vi "Kart_Pv_Emulator.vi"() -> ()   [LabVIEW 2016]
uses:
  <vilib>/Instr/_visa.llb/VISA Configure Serial Port (Instr).vi
  <vilib>/Utility/file.llb/Read From Spreadsheet File (DBL).vi
panel:
  out "error out":errorcluster
  out "Döngü Time":u32
  out "Veriler Grafiği":T1(graph)
  out "Model_I":dbl
  out "Model_V":dbl
  out "e_I":dbl
  out "e_V":dbl
  out "NuData":i32
  out "GucK_R":dbl
  out "PgucK":dbl=60.0
  out "Vi Panel":dbl
  out "GucK_W":dbl(knob) scale=0.0..60.0
  out "GucK_V":dbl(knob) scale=0.0..22.0
  in  "Port Sec":refnum<visa-resource-name>="COM1"
  out "GucK_I":dbl(knob) scale=0.0..3.7
  out "10_dk_ok":bool
  out "time":dbl
  out "i_Data":i32
  out "File patch":path
  out "Güç Grafiği":cluster{"PmaxM":dbl, "Pmaxe":dbl, "PgucK":dbl}(graph)
  in  "a":dbl=110.681443442253
  in  "Rs":dbl=25.0
  out "M_Pmax":dbl=60.29985558543294
  out "V - I Grafiği":cluster{"Vi":dbl, "Iint":dbl, dbl}(graph)={"Vi"=21.500000000000036, "Iint"=0.07178993987123095, 1.5434837072314678}
  in  "Rsh":dbl=110.681443442253
  in  "KV":dbl=-0.00863136
  in  "KI":dbl=0.0025624
  in  "ns":dbl=18.0
  out "e_Pmax":dbl=60.0
  in  "Voc":dbl=21.6
  in  "Isc":dbl=3.73
  in  "Vmp":dbl=17.3
  in  "Imp":dbl=3.47
  in  "G":dbl=1000.0
  in  "T":dbl=25.0
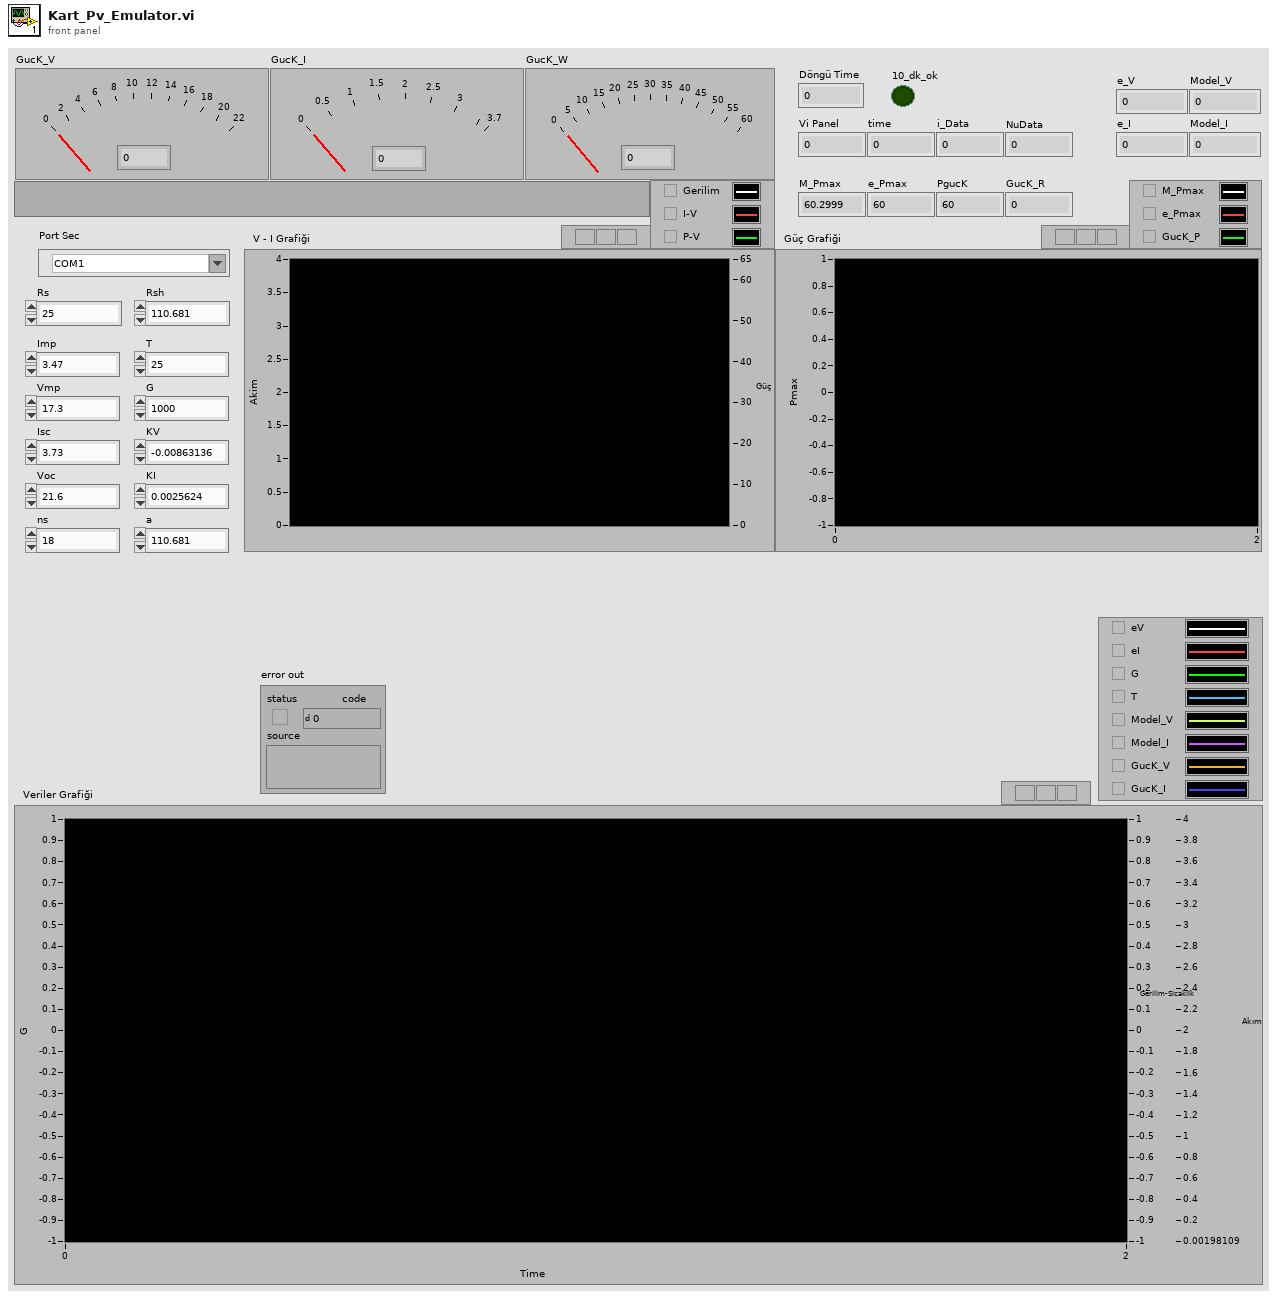
[diagram p1: front panel]
types:
  T1 = cluster{"e_V":dbl, "e_I":dbl, "G":dbl, "T":dbl, "Model_V":dbl, "Model_I":dbl, "GucK_V":dbl, "GucK_I":dbl}
  T2 = cluster{"e_V":dbl, "e_I":dbl, "G":dbl, "T":dbl, "Model_V":dbl, "Model_I":dbl, "GucK_V":dbl, "GucK_I":dbl}[]
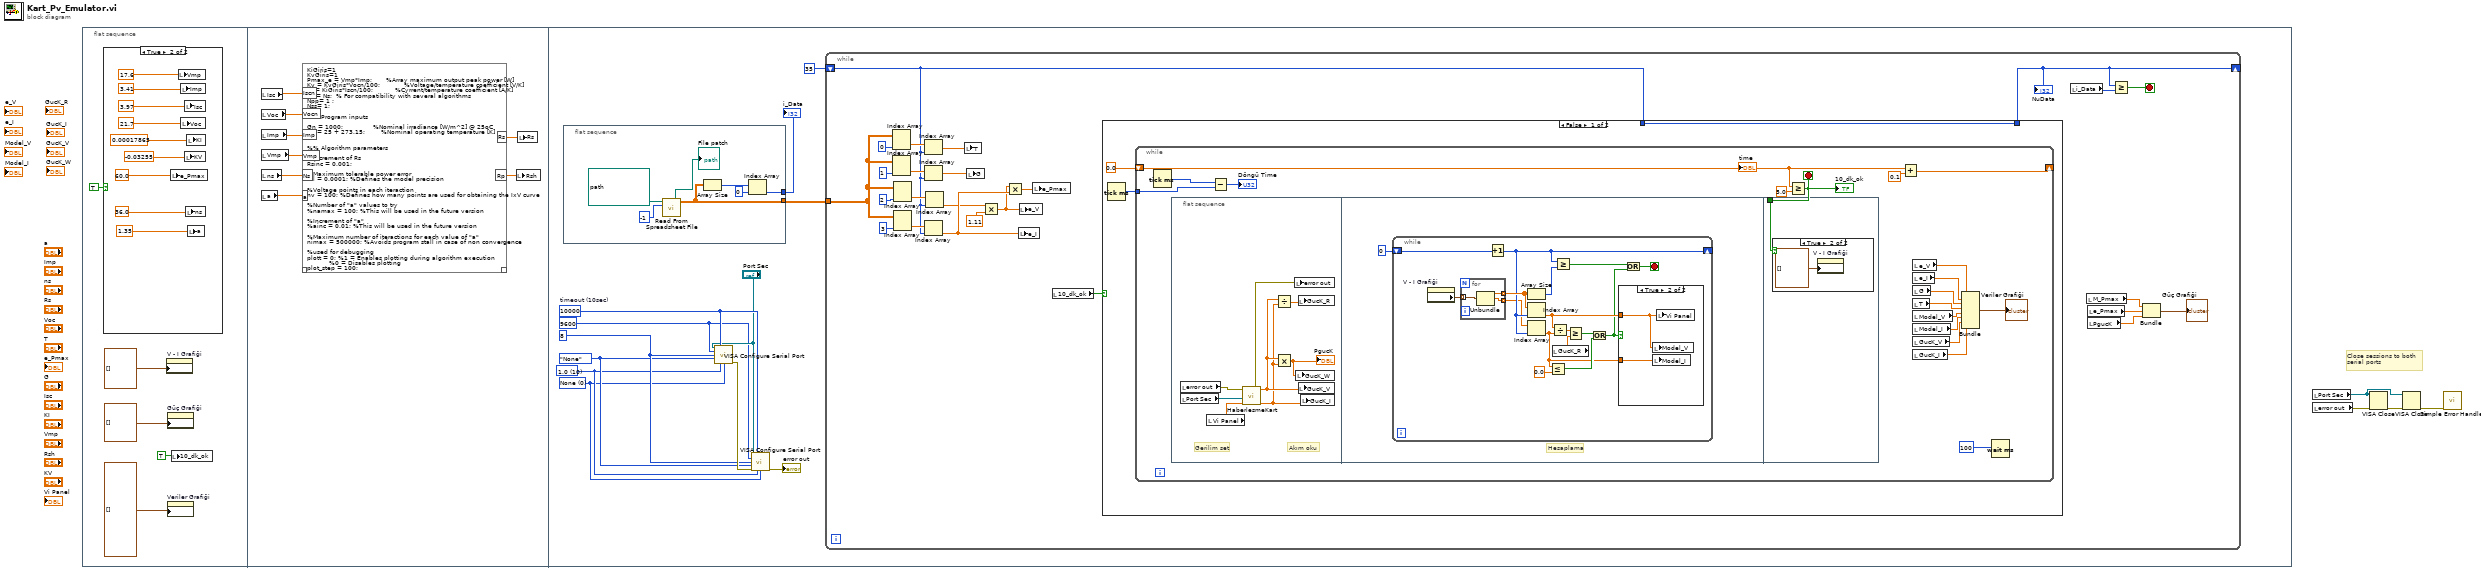
[diagram p0: block diagram]
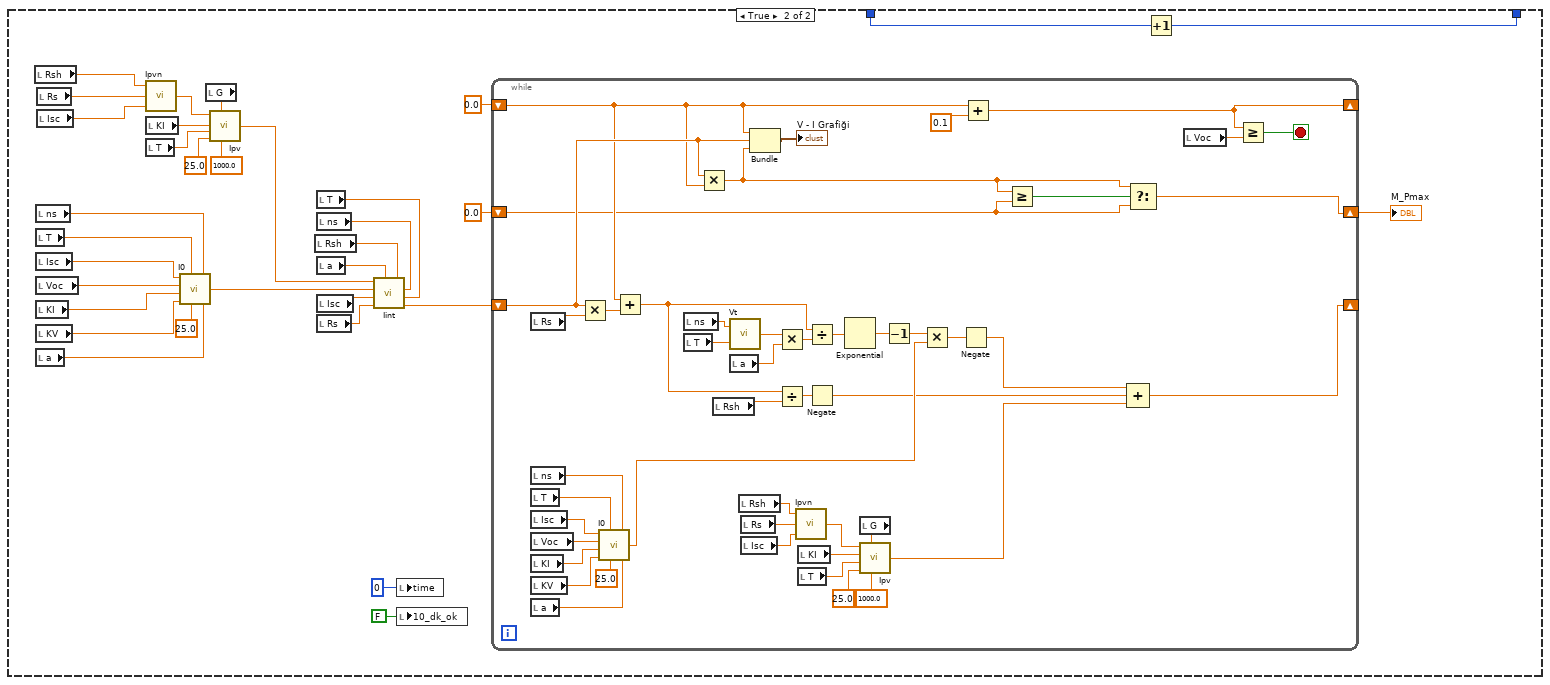
[diagram p5: hidden frame]
diagram:
  # "Close sessions to both serial ports"
  n1 = flat-sequence {
    frame #0 {
      n2 = case shown="True" TRUE {
        frame False {
        }
        frame True {
          n3 = local write "e_Pmax"(60.0 ("Pmaxe")) -> ()
          n4 = local write "Vmp"(17.6 ("Vmp")) -> ()
          n5 = local write "Imp"(3.41 ("Imp")) -> ()
          n6 = local write "Voc"(21.7 ("Voc")) -> ()
          n7 = local write "Isc"(3.97 ("Isc")) -> ()
          n8 = local write "KV"(-0.03255 ("KV")) -> ()
          n9 = local write "ns"(36.0 ("ns")) -> ()
          n10 = local write "KI"(0.00017865 ("KI")) -> ()
          n11 = local write "a"(1.35 ("ns")) -> ()
        }
      }
      n12 = property on="V - I Grafiği" class="WFChart (strict)"("History Data"=cluster{"Vi":dbl, "Iint":dbl, dbl}[] []) -> ()  [unwired: 2 in, 2 out]
      n13 = property on="Güç Grafiği" class="WFChart (strict)"("History Data"=cluster{"PmaxM":dbl, "Pmaxe":dbl, "PgucK":dbl}[] []) -> ()  [unwired: 2 in, 2 out]
      n14 = property on="Veriler Grafiği" class="WFChart (strict)"("History Data"=T2 []) -> ()  [unwired: 2 in, 2 out]
      n15 = local write "10_dk_ok"(TRUE ("10_dk_ok")) -> ()
    }
    frame #1 {
      n16 = local read "Isc"() -> (w22:dbl)
      n17 = local read "Voc"() -> (w19:dbl)
      n18 = local read "Imp"() -> (w23:dbl)
      n19 = local read "Vmp"() -> (w24:dbl)
      n20 = local read "ns"() -> (w25:dbl)
      n21 = local read "a"() -> (w26:dbl)
      n22 = script code="KiGiris=1\nKvGiris=1\nPmax_e = Vmp*Imp;       %Array maximum output peak power [W] \nKv = KvGiris*Vocn/100;            %Voltage/temperature coefficient [V/K] \nKi = KiGiris*Iscn/100;           %Cyrrent/temperature coefficient [A/K] \nns = Ns;  % For compatibility with several algorithms\nNpp= 1 ;\nNss= 1;\n \n%% Program inputs\n\nGn = 1000;               %Nominal irradiance [W/m^2] @ 25oC\nTn = 25 + 273.15;        %Nominal operating temperature [K]\n\n\n%% Algorithm parameters\n\n%Increment of Rs\nRsinc = 0.001;\n\n%Maximum tolerable power error\ntol = 0.0001; %Defines the model precision\n\n%Voltage points in each iteraction\nnv = 100; %Defines how many points are used for obtaining the IxV curve\n\n%Number of \"a\" values to try\n%namax = 100; %This will be used in the future version \n\n%Increment of \"a\"\n%ainc = 0.01; %This will be used in the future version \n\n%Maximum number of iteractions for each value of \"a\"\nnimax = 500000; %Avoids program stall in case of non convergence\n\n%used for debugging\nplott = 0; %1 = Enables plotting during algorithm execution\n           %0 = Disables plotting\nplot_step = 100;\n\n \n\n%% Adjusting algorithm\n\n% Reference values of Rs and Rp   \nRs_max = (Vocn - Vmp)/ Imp;\nRp_min = Vmp/(Iscn-Imp) - Rs_max;\n\n% Initial guesses of Rp and Rs\nRs = 0;\nRp = Rp_min;\n\n% The model is adjusted at the nominal condition\nT = Tn;\nG = Gn; \n\nk = 1.3806503e-23;   %Boltzmann [J/K]\nq = 1.60217646e-19;  %Electron charge [C]\n\nVtn = k * Tn / q;           %Thermal junction voltage (nominal) \nVt  = k * T  / q;           %Thermal junction voltage (current temperature)\n\n\nperror = Inf; %dummy value\n\n\n% Iterative process for Rs and Rp until Pmax,model = Pmax,experimental\n\nni = 0;\n\nwhile (perror>tol) && (Rp > 0) && (ni < nimax)\n\nni = ni + 1; \n    \n%  Temperature and irradiation effect on the current\ndT = T-Tn;\nIpvn = (Rs+Rp)/Rp * Iscn;         % Nominal light-generated current\nIpv = (Ipvn + Ki*dT) *G/Gn;       % Actual light-generated current \nIsc = (Iscn + Ki*dT) *G/Gn;       % Actual short-circuit current\n\nIo = (Ipv - Vocn/Rp)/(exp(Vocn/Vt/a/Ns)-1); %% NEW %% UPDATED ON JUNE/2010 %%\n\n% Increments Rs \nRs = Rs + Rsinc;  \n\nRp_ = Rp;\n\nRp = Vmp*(Vmp+Imp*Rs)/(Vmp*Ipv-Vmp*Io*exp((Vmp+Imp*Rs)/Vt/Ns/a)+Vmp*Io-Pmax_e);\n\n% Solving the I-V equation for several (V,I) pairs \n%clear V\n%clear I\n\nV = 0:Vocn/nv:Vocn;        % Voltage vector\nI = zeros(1,size(V,2));    % Current vector\n\nfor j = 1 : size(V,2) %Calculates for all voltage values \n    \n% Solves g = I - f(I,V) = 0 with Newton-Raphson\n  \ng(j) = Ipv-Io*(exp((V(j)+I(j)*Rs)/Vt/Ns/a)-1)-(V(j)+I(j)*Rs)/Rp-I(j);\n  \nwhile (abs(g(j)) > 0.001)\n      \ng(j) = Ipv-Io*(exp((V(j)+I(j)*Rs)/Vt/Ns/a)-1)-(V(j)+I(j)*Rs)/Rp-I(j);\nglin(j) = -Io*Rs/Vt/Ns/a*exp((V(j)+I(j)*Rs)/Vt/Ns/a)-Rs/Rp-1;\nI_(j) = I(j) - g(j)/glin(j);\nI(j) = I_(j);   \n  \nend  \n\nend % for j = 1 : size(V,2)\n\n%kapat\n%if (plott) \n    \n  %Plots the I-V and P-V curves\n\n  %Current x Voltage\n%  figure(1) \n% grid on\n%  hold on \n%  title('I-V curve - Adjusting Rs and Rp');\n%  xlabel('V [V]');\n%  ylabel('I [A]');\n%  xlim([0 Vocn]);\n%  ylim([0 Iscn]);\n \n  %Plots I x V curve\n%  plot(V,I,'LineWidth',2,'Color','k') \n \n  %Plots the \"remarkable points\" on the I x V curve\n%  plot([0 Vmp Vocn],[Iscn Imp 0],'o','LineWidth',2,'MarkerSize',5,'Color','k') \n\n  %Power x Voltage\n%  figure(2)  \n%  grid on\n%  hold on  \n%  title('P-V curve - Adjusting peak power');\n%  xlabel('V [V]');\n%  ylabel('P [W]');\n%  xlim([0 Vocn])\n%  ylim([0 Vmp*Imp]);\n    \n%end % if(plott)\n\n  % Calculates power using the I-V equation\n  P = (Ipv-Io*(exp((V+I.*Rs)/Vt/Ns/a)-1)-(V+I.*Rs)/Rp).*V;\n  \n  Pmax_m = max(P);\n  \n  perror = (Pmax_m-Pmax_e);\n\n%kapat  \n%if (plott) \n    \n  %Plots P x V curve\n%  plot(V,P,'LineWidth',2,'Color','k')\n  \n  %Plots the \"remarkable points\" on the power curve\n%  plot([0 Vmp Vocn],[0 Vmp*Imp 0],'o','LineWidth',2,'MarkerSize',5,'Color','k')\n  \n%end % if (plott)\n     \nend % while (error>tol) \n\nif (Rp<0) Rp = Rp_ \nend\n\nIon = Io; %\n\n\n%% Outputs\n \n % I-V curve\n% figure(3) \n% grid on\n% hold on \n% title('Adjusted I-V curve');\n% xlabel('V [V]');\n% ylabel('I [A]');\n% xlim([0 max(V)*1.1]);\n% ylim([0 max(I)*1.1]);\n \n% plot(V,I,'LineWidth',2,'Color','k') %\n% plot([0 Vmp Vocn ],[Iscn Imp 0 ],'o','LineWidth',2,'MarkerSize',5,'Color','k') \n \n % P-V curve\n\n% figure(4) \n% grid on\n% hold on \n% title('Adjusted P-V curve');\n% xlabel('V [V]');\n% ylabel('P [W]');\n% xlim([0 Vocn*1.1]);\n% ylim([0 Vmp*Imp*1.1]);\n  \n% plot(V,P,'LineWidth',2,'Color','k') %\n% plot([0 Vmp Vocn ],[0 Pmax_e 0 ],'o','LineWidth',2,'MarkerSize',5,'Color','k') \n   \n\n%disp(sprintf('Model info:\\n'));\n%disp(sprintf(' Rp_min = %f',Rp_min));\n%disp(sprintf('     Rp = %f',Rp));\n%disp(sprintf(' Rs_max = %f',Rs_max));\n%disp(sprintf('     Rs = %f',Rs));\n%disp(sprintf('      a = %f',a));\n%disp(sprintf('      T = %f',T-273.15));\n%disp(sprintf('      G = %f',G));\n%disp(sprintf(' Pmax,m = %f  (model)',Pmax_m));\n%disp(sprintf(' Pmax,e = %f  (experimental)',Pmax_e));\n%disp(sprintf('    tol = %f',tol));\n%disp(sprintf('P_error = %f',perror));\n%disp(sprintf('    Ipv = %f',Ipv));\n%disp(sprintf('    Isc = %f',Isc));\n%disp(sprintf('    Ion = %g',Ion));\n%disp(sprintf('    Ki = %g',Ki));\n%disp(sprintf('    Kv = %g',Kv));\n%disp(sprintf('\\n\\n'));\n\n\n%%% This feature is not available yet.\n%disp('Copy and paste this line of code in your simulation model:');\n%disp(sprintf('pvdata[14]={%f,%f,%f,%f,%f,%f,%f,%f,%f,%f,%f,%f,%f,%f};',Iscn,Vocn,Imp,Vmp,Kv,Ki,Ns,Gn,Tn,Rp,Rs,a,Ipvn,Ion));"("Iscn"=w22, "Vocn"=w19, "Imp"=w23, "Vmp"=w24, "Ns"=w25, "a"=w26) -> ("Rs"=w21:dbl, "Rp"=w20:dbl)  [unwired: 1 in, 1 out]
      n23 = local write "Rsh"(w20) -> ()
      n24 = local write "Rs"(w21) -> ()
    }
    frame #2 {
      w27 = u16 0 items=["None", "XON/XOFF", "RTS/CTS", "XON/XOFF & RTS/CTS", "DTR/DSR", "XON/XOFF & DTR/DSR"] ("flow control (0:none)")
      w28 = u16 10 items=["1.0"=10, "1.5"=15, "2.0"=20] ("stop bits (10: 1 bit)")
      w29 = enum16{"None", "Odd", "Even", "Mark", "Space"}."None" ("parity (0:none)")
      w30 = u16 8 ("data bits (8)")
      w31 = u32 9600 ("baud rate (9600)")
      w34 = u32 10000  # timeout (10sec)
      n25 = flat-sequence {
        tunnel: [w42] -> w36
        tunnel: [w39] -> w37
        frame #0 {
          n26 = call-poly <vilib>:"Read From Spreadsheet File.vi"("number of rows (all:-1)"=-1, "file path (dialog if empty)"=path "D:/YüksekLisans/Tez/uygula/Güneş Paneli Verileri/Tümü/Düzenlenen Veriler/Panel_6/P6Haziran29.xls") -> ("all rows"=w39:dbl[][], "new file path (Not A Path if cancelled)"=→"File patch":path)  [unwired: 2 in, 6 out]
          n27 = Array Size(array=w39) -> (size(s)=w43:i32[])
          n28 = Index Array(array=w43, index=0 ("index 2")) -> (element=w42:i32)
        }
      }
      n29 = call-poly "VISA Configure Serial Port"("VISA resource name"="Port Sec", "timeout (10sec)"=w34, "baud rate (9600)"=w31, "data bits (8)"=w30, "parity (0:none)"=w29, "stop bits (10: 1 bit)"=w28, "flow control (0:none)"=w27) -> ("error out"=w35:errorcluster)  [unwired: 2 in, 6 out]
      n30 = call-poly "VISA Configure Serial Port"("VISA resource name"="Port Sec", "timeout (10sec)"=w34, "baud rate (9600)"=w31, "data bits (8)"=w30, "parity (0:none)"=w29, "error in (no error)"=w35, "stop bits (10: 1 bit)"=w28, "flow control (0:none)"=w27) -> ("error out"=→"error out":errorcluster)  [unwired: 2 in, 5 out]
      n31 = while {
        shift-right: [w54] -> _
        shift-left: 35 -> [w53]
        tunnel: w37 -> [w58]
        stop <- w52 stop-if-true
        n32 = Index Array(array=w58, index (col)=0 ("disabled index (col)")) -> (element=w62:dbl[])  [unwired: 1 in]
        n33 = Index Array(array=w58, index (col)=1 ("disabled index (col)")) -> (element=w59:dbl[])  [unwired: 1 in]
        n34 = Index Array(array=w58, index (col)=2 ("disabled index (col)")) -> (element=w60:dbl[])  [unwired: 1 in]
        n35 = Index Array(array=w58, index (col)=3 ("disabled index (col)")) -> (element=w61:dbl[])  [unwired: 1 in]
        n36 = Index Array(array=w62, index=w53) -> (element=w56:dbl)
        n37 = Index Array(array=w59, index=w53) -> (element=w57:dbl)
        n38 = Index Array(array=w61, index=w53) -> (element=w50:dbl)
        n39 = Index Array(array=w60, index=w53) -> (element=w47:dbl)
        n40 = local write "T"(w56) -> ()
        n41 = local write "G"(w57) -> ()
        n42 = Multiply(x=w47, y=1.11) -> (x*y=w46:dbl)
        n43 = Multiply(x=w46, y=w50) -> (x*y=w48:dbl)
        n44 = local write "e_I"(w50) -> ()
        n45 = local write "e_V"(w46) -> ()
        n46 = local write "e_Pmax"(w48) -> ()
        n47 = local read "10_dk_ok"() -> (w55:bool)
        n48 = case shown="False" w55 {
          tunnel: [w72 w156] -> w54
          tunnel: w53 -> [w72 w155]
          frame False {
            n49 = Tick Count (ms)() -> (millisecond timer value=w71:u32)
            n50 = while {
              shift-right: [w89] -> _
              shift-left: 0.0 -> [w87]
              tunnel: w71 -> [w75]
              stop <- w88 stop-if-true
              n51 = Tick Count (ms)() -> (millisecond timer value=w74:u32)
              n52 = flat-sequence {
                tunnel: w88 -> [w122]
                frame #0 {
                  # "Gerilim set"
                  # "Akım oku"
                  n53 = local read "error out"() -> (w94:errorcluster)
                  n54 = local read "Port Sec"() -> (w92:refnum<visa-resource-name>)
                  n55 = local read "Vi Panel"() -> (w96:dbl)
                  n56 = call "HaberlesmeKart.vi"("error in (no error)"=w94, "VISA resource name"=w92, "Voltaj set"=w96) -> ("error out"=w93:errorcluster, "Voltaj"=w98:dbl, "Akım"=w95:dbl)  [unwired: 3 in]
                  n57 = Divide(x=w98, y=w95) -> (x/y=w99:dbl)
                  n58 = Multiply(x=w98, y=w95) -> (x*y=w97:dbl)
                  "PgucK" <- w97
                  n59 = local write "error out"(w93) -> ()
                  n60 = local write "GucK_W"(w97) -> ()
                  n61 = local write "GucK_R"(w99) -> ()
                  n62 = local write "GucK_V"(w98) -> ()
                  n63 = local write "GucK_I"(w95) -> ()
                }
                frame #1 {
                  # "Hesaplama"
                  n64 = while {
                    shift-right: [w111] -> _
                    shift-left: 0 -> [w114]
                    stop <- w107 stop-if-true
                    n65 = property on="V - I Grafiği" class="WFChart (strict)"() -> ("History Data"=w116:cluster{"Vi":dbl, "Iint":dbl, dbl}[])  [unwired: 2 in, 2 out]
                    n66 = for {
                      tunnel: w116 -> [w121] mode=indexing
                      tunnel: [w120] -> w115 mode=indexing
                      tunnel: [w119] -> w108 mode=indexing
                      n67 = Unbundle(w121) -> ("Vi"=w120:dbl, "Iint"=w119:dbl)  [unwired: 1 out]
                    }
                    n68 = Increment(x=w114) -> (x+1=w111:i32)
                    n69 = Array Size(array=w115) -> (size(s)=w113:i32)
                    n70 = Index Array(array=w115, index=w111) -> (element=w109:dbl)
                    n71 = Index Array(array=w108, index=w111) -> (element=w101:dbl)
                    n72 = Less Or Equal?(x=w101, y=0.0) -> (x <= y?=w104:bool)
                    n73 = Divide(x=w109, y=w101) -> (x/y=w110:dbl)
                    n74 = local read "GucK_R"() -> (w106:dbl)
                    n75 = Greater Or Equal?(x=w111, y=w113) -> (x >= y?=w112:bool)
                    n76 = Greater Or Equal?(x=w110, y=w106) -> (x >= y?=w103:bool)
                    n77 = Or(x=w103, y=w104) -> (x .or. y?=w102:bool)
                    n78 = case shown="True" w102 {
                      tunnel: w109 -> [_ w118]
                      tunnel: w101 -> [_ w117]
                      frame False {
                      }
                      frame True {
                        n79 = local write "Model_V"(w118) -> ()
                        n80 = local write "Model_I"(w117) -> ()
                        n81 = local write "Vi Panel"(w118) -> ()
                      }
                    }
                    n82 = Or(x=w112, y=w102) -> (x .or. y?=w107:bool)
                  }
                }
                frame #2 {
                  n83 = case shown="True" w122 {
                    frame False {
                    }
                    frame True {
                      n84 = property on="V - I Grafiği" class="WFChart (strict)"("History Data"=cluster{"Vi":dbl, "Iint":dbl, dbl}[] []) -> ()  [unwired: 2 in, 2 out]
                    }
                  }
                }
              }
              n85 = Subtract(x=w74, y=w75) -> (x-y=→"Döngü Time":u32)
              n86 = Greater Or Equal?(x=w87, y=5.0) -> (x >= y?=w88:bool)
              "10_dk_ok" <- w88
              n87 = Add(x=w87, y=0.1) -> (x+y=w89:dbl)
              n88 = local read "e_V"() -> (w78:dbl)
              n89 = local read "e_I"() -> (w79:dbl)
              n90 = local read "G"() -> (w80:dbl)
              n91 = local read "T"() -> (w81:dbl)
              n92 = local read "Model_V"() -> (w82:dbl)
              n93 = local read "Model_I"() -> (w83:dbl)
              n94 = local read "GucK_V"() -> (w84:dbl)
              n95 = local read "GucK_I"() -> (w85:dbl)
              n96 = Bundle("e_V"=w78, "e_I"=w79, "G"=w80, "T"=w81, "Model_V"=w82, "Model_I"=w83, "GucK_V"=w84, "GucK_I"=w85) -> (→"Veriler Grafiği":T1)  [unwired: 1 in]
              n97 = Wait (ms)(milliseconds to wait=u32 100 ("millisecond timer value")) -> ()  [unwired: 1 out]
              "time" <- w87
            }
          }
          frame True {
            n98 = local read "Rsh"() -> (w133:dbl)
            n99 = local read "ns"() -> (w145:dbl)
            n100 = local read "T"() -> (w146:dbl)
            n101 = local read "Isc"() -> (w147:dbl)
            n102 = local read "Voc"() -> (w148:dbl)
            n103 = local read "KI"() -> (w149:dbl)
            n104 = local read "KV"() -> (w150:dbl)
            n105 = local read "a"() -> (w129:dbl)
            n106 = local read "Rs"() -> (w127:dbl)
            n107 = local read "Isc"() -> (w144:dbl)
            n108 = call "Ipvn.vi"("Iscn"=w144, "Rs"=w127, "Rp"=w133) -> ("Ipvn"=w139:dbl)
            n109 = local read "KI"() -> (w142:dbl)
            n110 = local read "T"() -> (w143:dbl)
            n111 = call "I0.vi"("Iscn"=w147, "T"=w146, "Vocn"=w148, "KI"=w149, "Tn"=25.0, "KV"=w150, "ns"=w145, "a"=w129) -> ("I0"=w137:dbl)
            n112 = local read "G"() -> (w131:dbl)
            n113 = call "Ipv.vi"("Gn"=1000.0, "G"=w131, "Tn"=25.0, "T"=w143, "KI"=w142, "Ipvn"=w139) -> ("Ipv"=w138:dbl)
            n114 = local read "Rsh"() -> (w132:dbl)
            n115 = local read "T"() -> (w153:dbl)
            n116 = local read "ns"() -> (w152:dbl)
            n117 = local read "a"() -> (w128:dbl)
            n118 = local read "Isc"() -> (w136:dbl)
            n119 = local read "Rs"() -> (w130:dbl)
            n120 = call "Iint.vi"("T"=w153, "ns"=w152, "Rp"=w132, "a"=w128, "Rs"=w130, "Isc"=w136, "I0"=w137, "Ipv"=w138) -> ("Iint"=w154:dbl)
            n121 = local write "time"(u32 0 ("time")) -> ()
            n122 = local write "10_dk_ok"(FALSE ("10_dk_ok")) -> ()
            n123 = while {
              shift-right: [w158] -> _
              shift-left: 0.0 -> [w169]
              shift-right: [w179] -> _
              shift-left: w154 -> [w170]
              shift-right: [w167] -> w134
              shift-left: 0.0 -> [w166]
              stop <- w172 stop-if-true
              n124 = local read "Rs"() -> (w159:dbl)
              n125 = local read "ns"() -> (w197:dbl)
              n126 = local read "T"() -> (w196:dbl)
              n127 = local read "Isc"() -> (w195:dbl)
              n128 = local read "Voc"() -> (w194:dbl)
              n129 = local read "KI"() -> (w193:dbl)
              n130 = local read "KV"() -> (w192:dbl)
              n131 = local read "a"() -> (w160:dbl)
              n132 = Multiply(x=w170, y=w159) -> (x*y=w186:dbl)
              n133 = call "I0.vi"("Iscn"=w195, "T"=w196, "Vocn"=w194, "KI"=w193, "Tn"=25.0, "KV"=w192, "ns"=w197, "a"=w160) -> ("I0"=w181:dbl)
              n134 = Add(x=w169, y=w186) -> (x+y=w180:dbl)
              n135 = local read "ns"() -> (w188:dbl)
              n136 = local read "T"() -> (w189:dbl)
              n137 = Multiply(x=w170, y=w169) -> (x*y=w157:dbl)
              n138 = local read "Rsh"() -> (w165:dbl)
              n139 = call "Vt.vi"("T"=w189, "ns"=w188) -> ("Vt"=w187:dbl)
              n140 = local read "a"() -> (w161:dbl)
              n141 = local read "Rsh"() -> (w163:dbl)
              n142 = local read "Rs"() -> (w164:dbl)
              n143 = local read "Isc"() -> (w198:dbl)
              n144 = Bundle(w169, "Iint"=w170, w157) -> (→"V - I Grafiği":cluster{dbl, "Iint":dbl, dbl})  [unwired: 1 in]
              n145 = Multiply(x=w187, y=w161) -> (x*y=w185:dbl)
              n146 = Divide(x=w180, y=w165) -> (x/y=w174:dbl)
              n147 = call "Ipvn.vi"("Iscn"=w198, "Rs"=w164, "Rp"=w163) -> ("Ipvn"=w203:dbl)
              n148 = local read "KI"() -> (w200:dbl)
              n149 = local read "T"() -> (w199:dbl)
              n150 = Divide(x=w180, y=w185) -> (x/y=w184:dbl)
              n151 = Negate(x=w174) -> (-x=w175:dbl)
              n152 = Exponential(1:w184) -> (0:w183:dbl)
              n153 = local read "G"() -> (w162:dbl)
              n154 = call "Ipv.vi"("Gn"=1000.0, "G"=w162, "Tn"=25.0, "T"=w199, "KI"=w200, "Ipvn"=w203) -> ("Ipv"=w178:dbl)
              n155 = Decrement(x=w183) -> (x-1=w182:dbl)
              n156 = Multiply(x=w182, y=w181) -> (x*y=w177:dbl)
              n157 = Negate(x=w177) -> (-x=w176:dbl)
              n158 = Add(x=w169, y=0.1) -> (x+y=w158:dbl)
              n159 = Greater Or Equal?(x=w157, y=w166) -> (x >= y?=w168:bool)
              n160 = Compound Arithmetic op=ADD(w176, w175, w178) -> (w179:dbl)
              n161 = Select(t=w157, s=w168, f=w166) -> (s? t:f=w167:dbl)
              n162 = local read "Voc"() -> (w173:dbl)
              n163 = Greater Or Equal?(x=w158, y=w173) -> (x >= y?=w172:bool)
            }
            "M_Pmax" <- w134
            n164 = Increment(x=w155) -> (x+1=w156:i32)
          }
        }
        "NuData" <- w54
        n165 = local read "i_Data"() -> (w70:i32)
        n166 = local read "M_Pmax"() -> (w68:dbl)
        n167 = local read "e_Pmax"() -> (w67:dbl)
        n168 = local read "PgucK"() -> (w51:dbl)
        n169 = Greater Or Equal?(x=w54, y=w70) -> (x >= y?=w52:bool)
        n170 = Bundle("M_Pmax"=w68, "e_Pmax"=w67, "PgucK"=w51) -> (→"Güç Grafiği":cluster{"M_Pmax":dbl, "e_Pmax":dbl, "PgucK":dbl})  [unwired: 1 in]
      }
      "i_Data" <- w36
    }
  }
  n171 = local read "Port Sec"() -> (w1:refnum<visa-resource-name>)
  n172 = local read "error out"() -> (w2:errorcluster)
  n173 = VISA Close(VISA resource name=w1, error in (no error)=w2) -> (error out=w3:errorcluster)
  n174 = VISA Close(VISA resource name=w1, error in (no error)=w3) -> (error out=w4:errorcluster)
  n175 = call <vilib>:"Simple Error Handler.vi"("error in (no error)"=w4) -> ()  [unwired: 1 in, 8 out]
